vi "SetGagePrams.vi"(4 "Pts to take":i32=1000, 8 "Time scale per Div":i32(ring)=3 items=["100 ns", "200 ns", "500 ns", "1 micros", "2 micros", "5 micros", "10 micros", "20 micros", "50 micros", "100 micros", "500 micros", "1 ms", "5 ms", "10 ms"], 10 "Channel":u16(ring) items=["Ch 0", "Ch 1"], 11 "RF data Sampling":T2={"Sampling Rate"=50, "Ref Delay (ms)"=0.0, "rf points per line"=2500} {"Ref Delay (ms)" format="%.2f"}) -> (0 "Time per division":dbl format="%.2f", 2 "sampling rate":dbl, 3 "Temp Set Up Digi Params":T1)   [LabVIEW 2022 SP3]
uses:
  ProstateDataAcq/-ProstateScanSystem/RFSamplingCluster.ctl
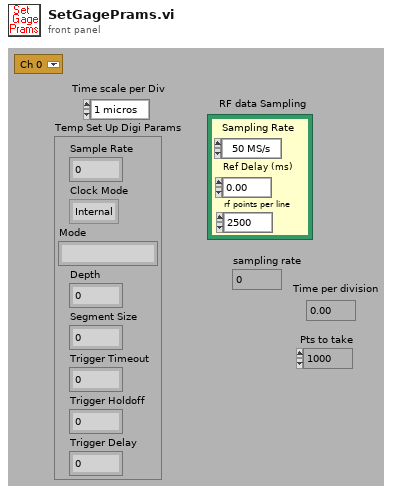
[diagram p1: front panel]
types:
  T1 = cluster{"Sample Rate":dbl, "Clock Mode":enum16{"Internal", "External", "Reference"}, "Mode":string, "Depth":dbl, "Segment Size":dbl, "Trigger Timeout":dbl, "Trigger Holdoff":dbl, "Trigger Delay":dbl}
  T2 = typedef "RFSamplingCluster.ctl" = cluster{"Sampling Rate":u16, "Ref Delay (ms)":dbl, "rf points per line":u16}
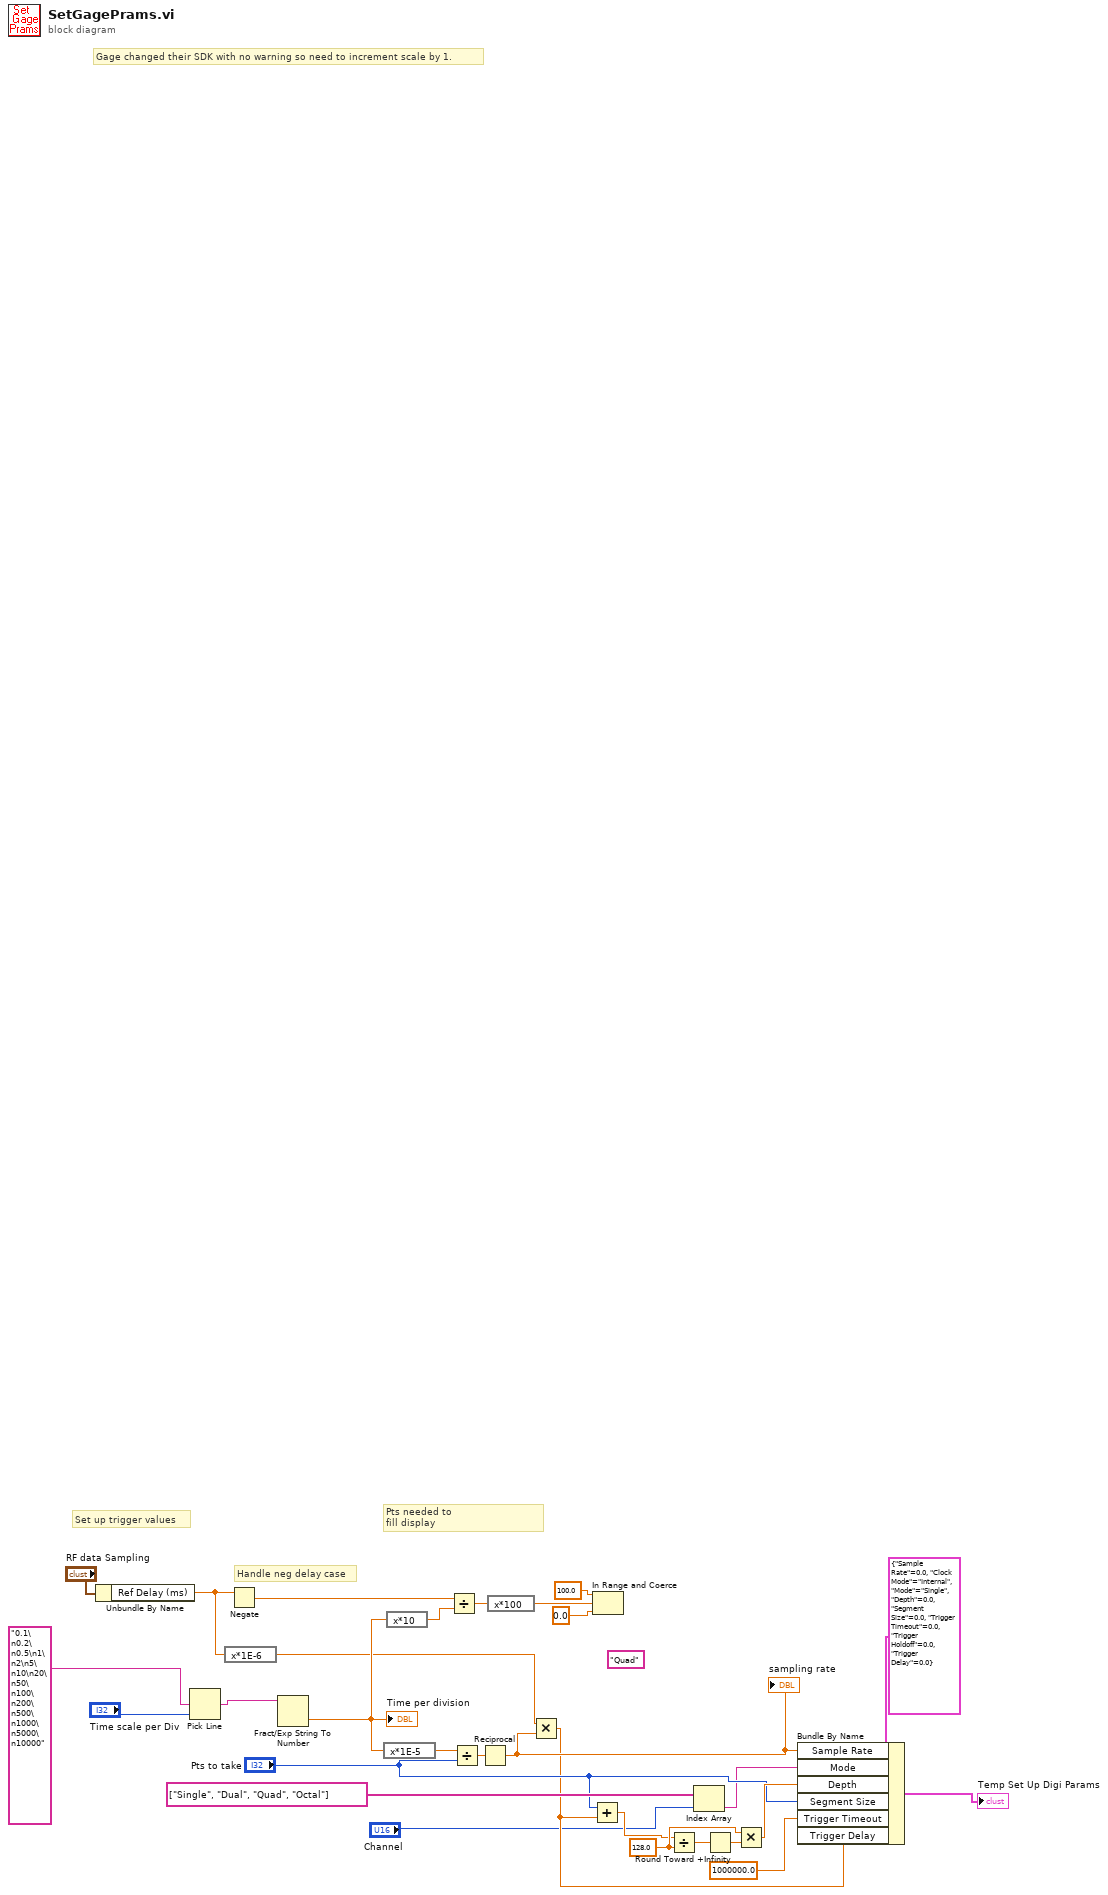
[diagram p0: block diagram]
diagram:
  (unwired) "Quad"
  w8 = 128.0 ("y")
  # "Handle neg delay case"
  # "Pts needed to\nfill display"
  # "Set up trigger values"
  # "Gage changed their SDK with no warning so need to increment scale by 1."
  n1 = Unbundle By Name("RF data Sampling") -> ("Ref Delay (ms)"=w12:dbl)
  n2 = Pick Line(multi-line string="0.1\n0.2\n0.5\n1\n2\n5\n10\n20\n50\n100\n200\n500\n1000\n5000\n10000" ("ResourceName"), line index="Time scale per Div") -> (output string=w6:string)  [unwired: 1 out]
  n3 = expression code="x*1E-6"(w12) -> (w11:dbl)
  n4 = Negate(x=w12) -> (-x=w14:dbl)
  n5 = Fract/Exp String To Number(string=w6) -> (number=w15:dbl)  [unwired: 1 in, 3 out]
  "Time per division" <- w15
  n6 = expression code="x*1E-5"(w15) -> (w20:dbl)
  n7 = expression code="x*10"(w15) -> (w21:dbl)
  n8 = Divide(x=w14, y=w21) -> (x/y=w22:dbl)
  n9 = Divide(x=w20, y="Pts to take") -> (x/y=w19:dbl)
  n10 = Reciprocal(x=w19) -> (1/x=w13:dbl)
  "sampling rate" <- w13
  n11 = expression code="x*100"(w22) -> (w23:dbl)
  n12 = Multiply(x=w11, y=w13) -> (x*y=w3:dbl)
  n13 = Add(x="Pts to take", y=w3) -> (x+y=w4:dbl)
  n14 = In Range and Coerce(upper limit=100.0, x=w23, lower limit=0.0) -> ()  [unwired: 2 out]
  n15 = Divide(x=w4, y=w8) -> (x/y=w10:dbl)
  n16 = Index Array(array=string[] ["Single", "Dual", "Quad", "Octal"], index="Channel") -> (element=w2:string)
  n17 = Round Toward +Infinity(x=w10) -> (ceil(x): smallest int >= x=w9:dbl)
  n18 = Multiply(x=w8, y=w9) -> (x*y=w7:dbl)
  n19 = Bundle By Name(cluster=T1 {"Sample Rate"=0.0, "Clock Mode"=enum."Internal", "Mode"="Single", "Depth"=0.0, "Segment Size"=0.0, "Trigger Timeout"=0.0, "Trigger Holdoff"=0.0, "Trigger Delay"=0.0} ("Acquisition"), "Sample Rate"=w13, "Mode"=w2, "Depth"=w7, "Segment Size"="Pts to take", "Trigger Timeout"=1000000.0, "Trigger Delay"=w3) -> (→"Temp Set Up Digi Params":T1)
